vi "sub_img_process.vi"(8 "error in":errorcluster, 10 "Green or Sat Plane":T1, 11 "Image Src":T1) -> (0 "error out":errorcluster, 3 "Image Dst Out":T1)   [LabVIEW 2019]
uses:
  <vilib>/vision/Image Controls.llb/IMAQ Image.ctl
  <vilib>/vision/NI_Vision_Development_Module.lvlib
panel:
  out "Image 2":T1(plugin-control)
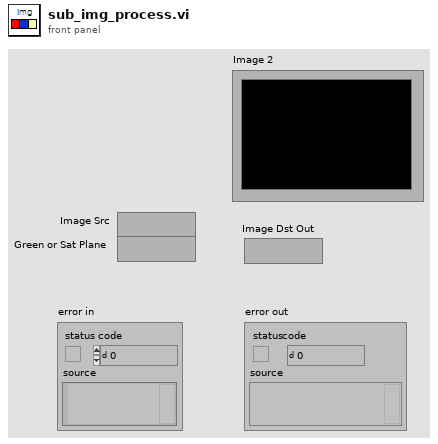
[diagram p1: front panel]
types:
  T1 = typedef "IMAQ Image.ctl" = refnum<image>
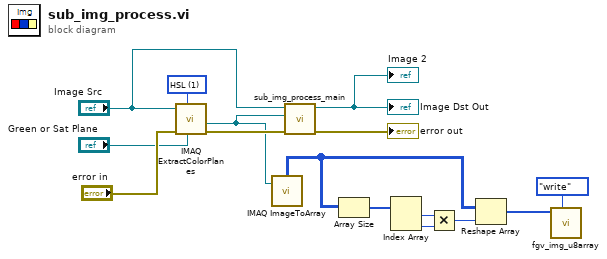
[diagram p0: block diagram]
diagram:
  w15 = u16 1 items=["RGB", "HSL", "HSV", "HSI"] ("Color Mode")
  n1 = call "IMAQ ExtractColorPlanes"("Blue or Luma or Val or Inten Plane"="Green or Sat Plane", "Color Mode"=w15, "error in (no error)"="error in", "Image Src"="Image Src") -> ("error out"=w14:errorcluster, "Blue or Luma or Val or Inten Plane out"=w8:T1)  [unwired: 4 in, 2 out]
  n2 = call "IMAQ ImageToArray"("Image"=w8) -> ("Image Pixels (U8)"=w6:u8[][])  [unwired: 3 in, 4 out]
  n3 = call "sub_img_process_main.vi"("error in"=w14, "Image Dst"=w8, "Image Src"="Image Src") -> ("error out"=→"error out":errorcluster, "Image roi-in"=→"Image Dst Out" →"Image 2":T1)  [unwired: 5 in, 2 out]
  n4 = Array Size(array=w6) -> (size(s)=w4:i32[])
  n5 = Index Array(array=w4) -> (element #1=w2:i32, element #2=w3:i32)  [unwired: 2 in]
  n6 = Multiply(x=w2, y=w3) -> (x*y=w1:i32)
  n7 = Reshape Array(w6, w1) -> (w5:u8[])
  n8 = call "fgv_img_u8array.vi"("cmd"=enum16{"init", "read", "write"}."write", "data"=w5) -> ()  [unwired: 9 in, 1 out]
